vi "closeFile.vi"(8 "error in (no error)":errorcluster, 11 "reference in":refnum<class "excelFile.lvclass">) -> (0 "error out":errorcluster, 3 "reference out":refnum<class "excelFile.lvclass">)   [LabVIEW 2015, in "excelFile.lvclass"]
uses:
  excelFile.lvclass
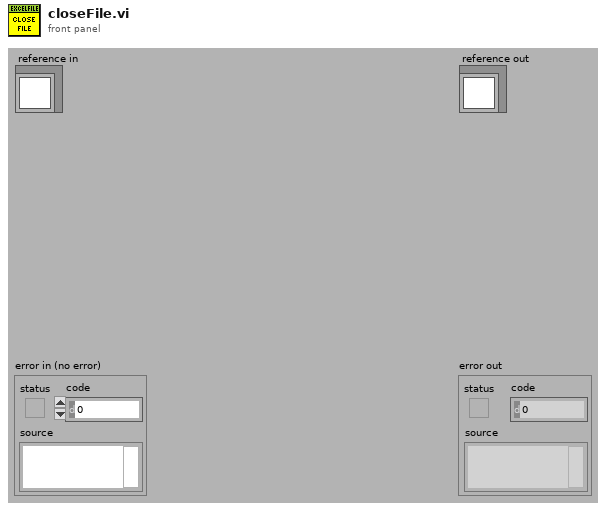
[diagram p1: front panel]
types:
  T1 = typedef "excelFile.lvclass/ObjectAttributesRef.ctl" = refnum<data-value>
  T2 = typedef "excelFile.lvclass/ObjectAttributes.ctl" = cluster{"MyAttribute":dbl, "path":string, "Refnum Excel":cluster{"Excel._Application":refnum<k7>, "Workbooks":refnum<k7>, "Open":refnum<k7>}, "data":string[][][], "fileType":T3, "sheetName":string[]}
  T3 = typedef "excelFile.lvclass/fileType.ctl" = enum16{"database", "CosmedTest"}
  T4 = cluster{"Excel._Application":refnum<k7>, "Workbooks":refnum<k7>, "Open":refnum<k7>}
  T5 = cluster{"Excel._Application":refnum<k7>, "Workbooks":refnum<k7>}
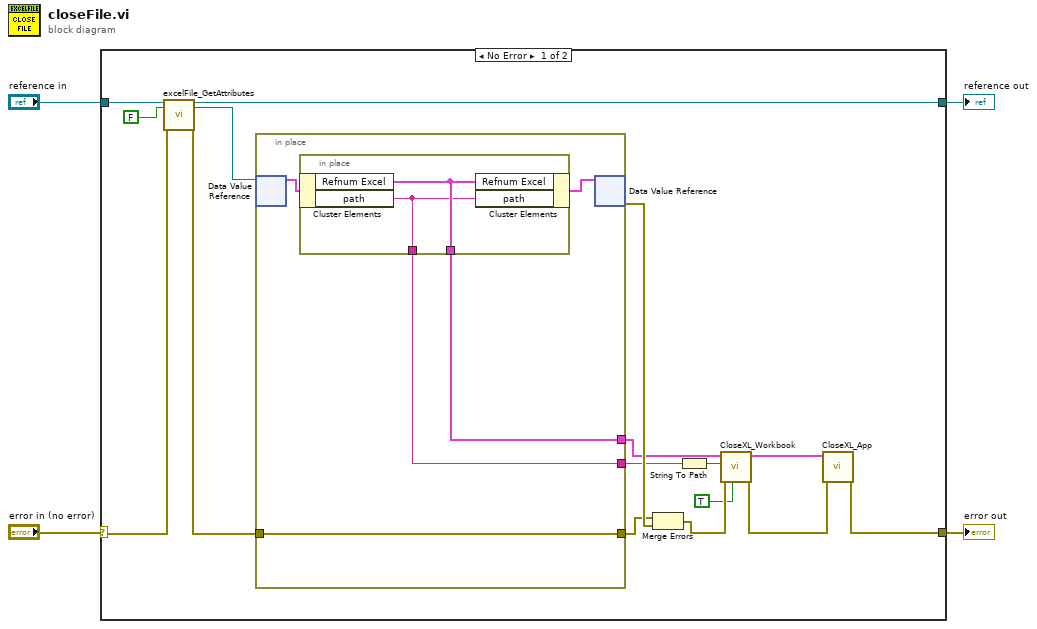
[diagram p0: block diagram]
diagram:
  n1 = case shown="No Error" "error in (no error)" {
    selector: "error in (no error)" -> [w16 w29]
    tunnel: [w8 w29] -> w3
    tunnel: [w14 w28] -> w1
    tunnel: "reference in" -> [w18 w28]
    frame No Error {
      n2 = call "excelFile_GetAttributes.vi"("reference in"=w18, "return data? (T)"=FALSE, "error in (no error)"=w16) -> ("reference out"=w14:refnum<class "excelFile.lvclass">, "attributes ref"=w13:T1, "error out"=w15:errorcluster)  [unwired: 13 in, 1 out]
      n3 = in-place {
        in-place-border: w15 -> [w23]
        in-place-border: [w23] -> w19
        in-place-border: [w22] -> w11
        in-place-border: [w21] -> w6
        n4 = in-place-dvr #1(w13) -> (w24:T2)  [unwired: 1 out]
        n5 = in-place {
          in-place-border: [w27] -> w22
          in-place-border: [w26] -> w21
          n6 = in-place-cluster #2(w24) -> ("Refnum Excel"=w27:T4, "path"=w26:string)
          n7 = in-place-cluster #2("Refnum Excel"=w27, "path"=w26) -> (w25:T2)
        }
        n8 = in-place-dvr #1(w25) -> (w20:errorcluster)  [unwired: 1 out]
      }
      n9 = Merge Errors(w19, w20) -> (w12:errorcluster)
      n10 = String To Path(string=w6) -> (path=w5:path)
      n11 = call <userlib>:"CloseXL_Workbook.vi"("Save? (F)"=TRUE, "error in (no error)"=w12, "path"=w5, "Refnum Cluster In"=w11) -> ("error out"=w9:errorcluster, "Refnum Cluster Out"=w10:T5)  [unwired: 6 in]
      n12 = call <userlib>:"CloseXL_App.vi"("error in (no error)"=w9, "Refnum Cluster In"=w10) -> ("error out"=w8:errorcluster)  [unwired: 9 in]
    }
    frame Error {
    }
  }
  "error out" <- w3
  "reference out" <- w1
